vi "Set separate class.vi"() -> ()   [LabVIEW 2015]
panel:
  in  "Stop on bad":bool=TRUE
  out "Modified files":path[](array[path])
  out "Modified":i32
  in  "Stop Button":bool
  out "File Path":path
  out "Progress":string
  in  "Folder Path":path
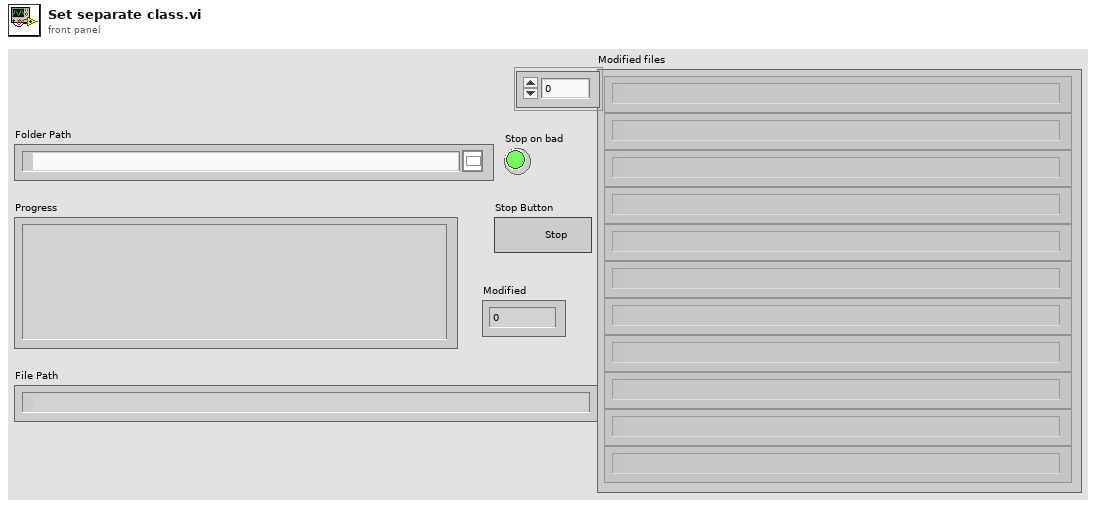
[diagram p1: front panel]
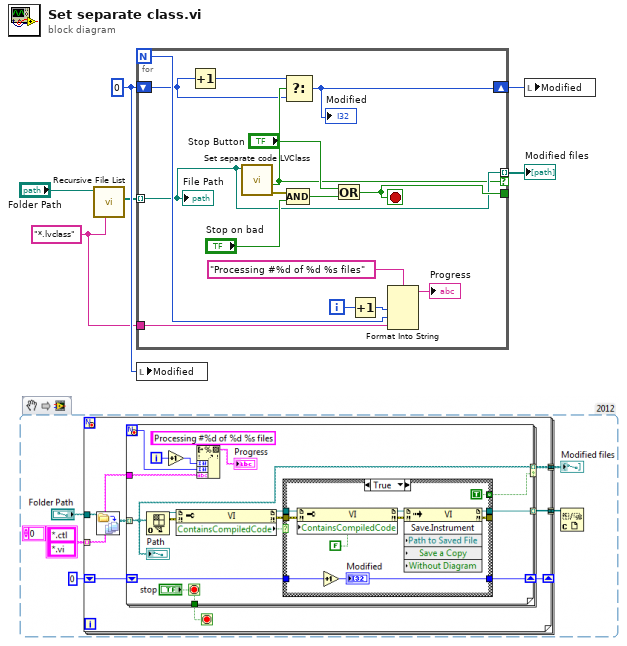
[diagram p0: block diagram]
diagram:
  w2 = "*.lvclass"
  w4 = 0 ("Modified")
  n1 = call <vilib>:"Recursive File List.vi"("pattern"=w2, "Folder Path"="Folder Path") -> ("All Files in Dir"=w3:path[])  [unwired: 5 in, 4 out]
  n2 = for {
    N -> [w19]
    tunnel: w3 -> [w12] mode=indexing
    tunnel: w2 -> [w18]
    tunnel: [w14] -> _
    shift-right: [w7] -> w1
    shift-left: w4 -> [w8]
    tunnel: [w12] -> w5 mode=indexing if=w10
    i -> [w21]
    stop <- w14 stop-if-true
    n3 = Increment(x=w8) -> (x+1=w9:i32)
    n4 = call "Set separate code LVClass.vi"("File Path"=w12) -> ("error out"=w11:errorcluster, "Saved"=w10:bool)  [unwired: 8 in, 1 out]
    n5 = Select(t=w9, s=w10, f=w8) -> (s? t:f=w7:i32)
    "Modified" <- w7
    n6 = Compound Arithmetic op=AND(w11, "Stop on bad") -> (w13:bool)
    n7 = Or(x="Stop Button", y=w13) -> (x .or. y?=w14:bool)
    n8 = Increment(x=w21) -> (x+1=w20:i32)
    n9 = Format Into String(format string="Processing #%d of %d %s files", w20, w19, w18) -> (resulting string=→"Progress":string)  [unwired: 2 in, 1 out]
    "File Path" <- w12
  }
  "Modified files" <- w5
  n10 = local write "Modified"(w4) -> ()
  n11 = local write "Modified"(w1) -> ()
